vi "close.vi"(0 "reference":refnum<class "OSA.lvclass">, 5 "error in (no error)":errorcluster) -> (19 "error out":errorcluster)   [LabVIEW 2010, in "OSA.lvclass"]
uses:
  OSA.lvclass
  OSA.lvclass/OSA.ctl
  FTSLib.dll
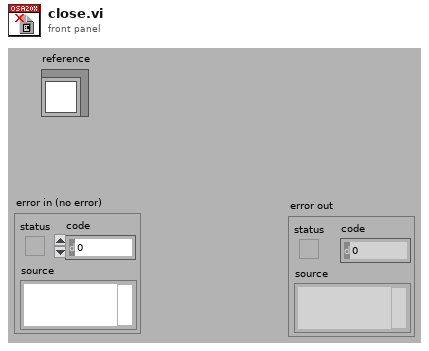
[diagram p1: front panel]
types:
  T1 = typedef "OSA.lvclass/ObjectAttributes.ctl" = cluster{"Stop":bool, "dataType":T2, "spectrometerIdx":u16, "buffer size interferogram":i32, "interferogram":cluster{"new":bool, "plot_x_ min":sgl, "plot_x_max":sgl, "plot_y_min":sgl, "plot_y_max":sgl, "Graph Intrfrgrm":T3, "timeStamp":u32, "signal (%)":dbl, "traces":cluster{"idx":u32, "broadBand":bool, "monoChromatic":bool, "peakToPeakSignal":dbl, "peakToPeakPos":dbl}[], "traces idx last":i32}, "spectrum":cluster{"new":bool, "plot_x_min":sgl, "plot_x_max":sgl, "plot_unit_x":T4, "plot_unit_y":T5, "plot_y_min":sgl, "plot_y_max":sgl, "Graph Spectrum":T3, "timeStamp":u32, "X_VAL_OPTIONS":enum16{"MIN_MAX", "ARRAY"}, "traces":cluster{"idx":u32}[], "traces idx last":i32}, "Thorlabs_OSA_64.lvclass:queue_action.ctlqueue ref":refnum<queue>, "action":T6, "plot zoom step":dbl, "buffer semaphore":T7, "acq stopped":bool, "dataType active":T2, "temperature (degr C)":sgl, "pressure (hPa)":sgl, "rel humidity (%)":sgl, "settings":cluster{"resolution":T8, "sensitivity":T9, "Average":bool, "average nr":u32, "apodisation":T10, "acq delay (ms)":u32, "airMesure":T11, "wmtr on":bool, "intfgrm_smooth_width":u16, "intfgrm_smooth_nrOfPasses":u16, "intfgrm_smooth":T12, "phaseCorrection":T13, "zeroFill":u8, "spectr_smooth":T12, "spectr_smooth_width":u16, "spectr_smooth_nrOfPasses":u16, "resolution (/cm)":sgl, "REF wavelength, (nm)":dbl, "gain_idx":u16, "gainAuto":bool, "gain_relative":dbl, "PD sensitivity mode":T14, "PD senseMode implemented":bool, "SensorTemperature implemented":bool, "SensorPressure implemented":bool, "SensorHumidity implemented":bool}, "peaks position":sgl[], "peaks width":sgl[], "peaks height":sgl[], "peaks max nr":u32, "peaks latest nr":i32, "peaks new":bool, "power":dbl, "power new":bool, "path":string, "wavelength (WNr)":dbl, "wavelength new":bool, "buffer size spectrum":i32, "status":string, "VI reference":refnum<vi>, "funcPointer":u64, "libraryPointer":u64, "singleAcquisition":bool, "coherenceLength (cm)":dbl, "coherenceLength new":bool, "spectrometer model":string, "spectrometer serial nr":string, "peaks thld left":sgl[], "peaks thld right":sgl[], "coherenceLength error (cm)":dbl, "ADC bits":u16, "peaks position centroid":sgl[], "peaks height centroid":sgl[], "OSA series":T15, "channel index (all)":u16}
  T2 = typedef "OSA.lvclass/acq_dataType.ctl" = enum16{"none", "interferogram", "spectrum"}
  T3 = typedef "OSA.lvclass/graph_intensity.ctl" = refnum<vi>
  T4 = typedef "OSA.lvclass/spectrum_x_unit.ctl" = enum16{"wavenr/cm", "THz", "eV", "nm_air", "nm_vac"}
  T5 = typedef "OSA.lvclass/y_unit.ctl" = enum16{"ADC counts", "dBm pwr absolute", "dBm pwr density", "mW pwr absolute", "mW pwr density"}
  T6 = typedef "OSA.lvclass/queue_action.ctl" = enum16{"none", "stop", "GUI_plotInterferogram", "GUI_plotSpectrum", "GUI_plotInterferogramRescale", "GUI_plotSpectrumRescale", "GUI_plotInterferogramReset", "GUI_plotSpectrumReset", "GUI_plotInterferogramAutoScaleY", "GUI_plotSpectrumAutoScaleY", "GUI_plotInterferogramZoomOut", "GUI_plotSpectrumZoomOut", "GUI_plotInterferogramPane", "GUI_plotSpectrumPane", "GUI_plotInterferogramZoomMouse", "GUI_plotSpectrumZoomMouse", "ENVIRONMENT temperature", "ENVIRONMENT pressure", "MODE_resolution set", "MODE_resolution get", "MODE_sensitivity set", "MODE_sensitivity get", "MODE_PDTemperature set", "MODE_PDTemperature get", "REBOOT/RESET firmware", "ACQASYNC_acquireSingleSpectrum", "ACQASYNC_continuous start", "ACQASYNC_continuous stop\n", "ACQASYNC_get last interferogram", "ACQASYNC_get last spectrum", "ACQASYNC_get last waveNr", "ACQOPT_interferogram smoothing set", "ACQOPT_interferogram smoothing get", "ACQOPT_spectrum smoothing set", "ACQOPT_spectrum smoothing get", "ACQOPT_apodisation type set", "ACQOPT_apodisation type get", "ACQOPT_phase correction type set", "ACQOPT_phase correction type get", "ACQOPT_acqIntervall_set", "ACQOPT_acqIntervall_get", "ACQOPT_average spectrum set", "ACQOPT_average spectrum get", "ACQOPT_rolling average set", "ACQOPT_rolling average get", "ACQOPT_zero fill factor set", "ACQOPT_zero fill factor get", "ACQOPT_cycle counting set", "ACQOPT_cycle counting get", "ACQOPT_air measure option set", "ACQOPT_air measure option get", "ACQOPT_gainLevel auto get", "ACQOPT_gainLevel auto set", "ACQOPT_gainLevel get", "ACQOPT_gainLevel set", "ACQOPT_getAll", "INSTRUMENT_PROPERTY_range_WaveNr_min", "INSTRUMENT_PROPERTY_range_WaveNr_max", "INSTRUMENT_PROPERTY_reference_wavelength_cm^-1", "INSTRUMENT_PROPERTY_samplesPerRefPeriod", "INSTRUMENT_PROPERTY_resolution_waveNrPercm", "INSTRUMENT_PROPERTY_availableGainLevels", "INSTRUMENT_PROPERTY_status", "CONVERT", "ANALYSE_POWER", "ANALYSE_PEAKS", "ANALYSE_WAVELENGTH", "ANALYSE_SPECTRUM", "ANALYSE_INTERFEROGRAM", "ANALYSE_COHERENCE_LENGTH", "MATH", "MATH_power", "MATH_peaks", "FILE", "miscellaneous"}
  T7 = typedef "Semaphore RefNum" = refnum<k1>
  T8 = typedef "OSA.lvclass/resolution.ctl" = enum16{"low", "high"}
  T9 = typedef "OSA.lvclass/sensitivityMode.ctl" = enum16{"low", "low medium", "high medium", "high"}
  T10 = typedef "OSA.lvclass/apodisation.ctl" = enum16{"NONE", "NORTON_BEER_WEAK", "NORTON_BEER_MEDIUM", "NORTON_BEER_STRONG", "TRIANGULAR", "COSINE", "HANN", "HAMMING", "BLACKMANHARRIS3", "BLACKMANHARRIS4", "GAUSSIAN"}
  T11 = typedef "OSA.lvclass/airMeasure.ctl" = enum16{"TEMPERATURE", "PRESSURE"}
  T12 = typedef "OSA.lvclass/smoothing.ctl" = enum16{"NONE", "BINOMIAL", "SAVITSKY_GOLAY", "FOURIER", "MOVING_AVERAGE", "GAUSSIAN"}
  T13 = typedef "OSA.lvclass/phaseCorrection.ctl" = enum16{"NONE", "MERTZ", "FORMAN", "MERTZ_FILE", "FORMAN_FILE", "FUTURE COMP."}
  T14 = typedef "OSA.lvclass/PDTemperatureMode.ctl" = enum16{"cool: better sensitivity/noise floor", "warm: extended wl range"}
  T15 = typedef "OSA_series.ctl" = enum16{"OSA200", "OSA300", "UNKNOWN"}
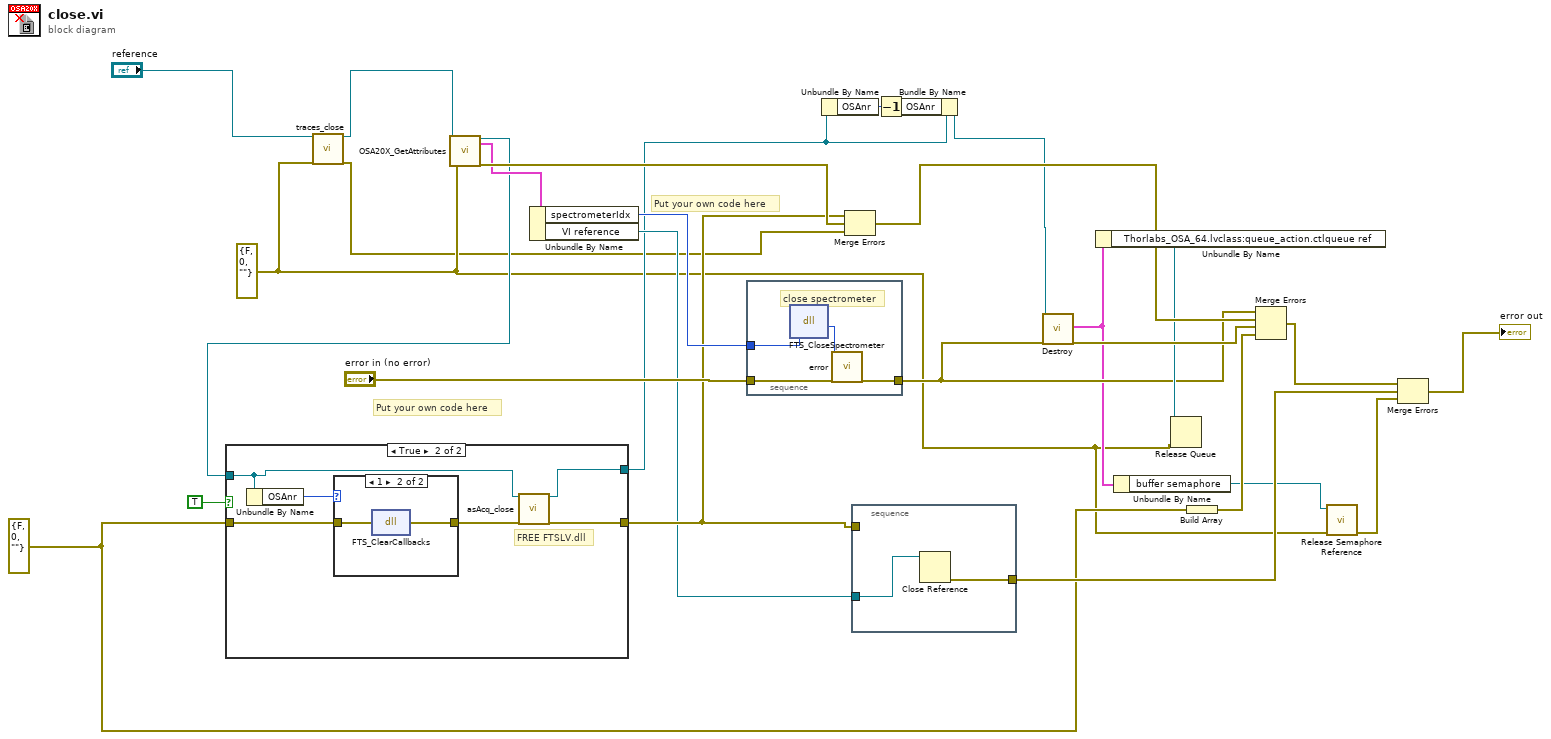
[diagram p0: block diagram]
diagram:
  w15 = errorcluster {"status"=FALSE, "code"=0, "source"=""} ("error in")
  w2 = errorcluster {"status"=FALSE, "code"=0, "source"=""} ("error in (no error)")
  # "Put your own code here"
  # "Put your own code here"
  n1 = call "traces_close.vi"("reference"="reference", "error in (no error)"=w2) -> ("duplicate reference"=w3:refnum<class "OSA.lvclass">, "error out"=w1:errorcluster)  [unwired: 16 in]
  n2 = call "OSA20X_GetAttributes.vi"("reference in"=w3, "error in (no error)"=w2) -> ("reference out"=w12:refnum<class "OSA.lvclass">, "Data"=w14:T1, "error out"=w22:errorcluster)  [unwired: 14 in, 1 out]
  n3 = case shown="True" TRUE {
    tunnel: w12 -> [w30 w31]
    tunnel: [w30 w36] -> w11
    tunnel: [w29 w35] -> w20
    tunnel: w15 -> [w29 w34]
    frame False {
    }
    frame True {
      # "FREE FTSLV.dll"
      n4 = Unbundle By Name(w31) -> ("OSAnr"=w32:i32)
      n5 = case shown="1" w32 {
        tunnel: w34 -> [w37 w39]
        tunnel: [w37 w38] -> w33
        frame 0, Default {
        }
        frame 1 {
          n6 = dll-call lib="FTSLib.dll" fn="FTS_ClearCallbacks"(error in=w39) -> (error out=w38:errorcluster)  [unwired: 3 in, 1 out]
        }
      }
      n7 = call "asAcq_close.vi"("reference"=w31, "error in (no error)"=w33) -> ("duplicate reference"=w36:refnum<class "OSA.lvclass">, "error out"=w35:errorcluster)  [unwired: 16 in]
    }
  }
  n8 = Unbundle By Name(w14) -> ("spectrometerIdx"=w27:u16, "VI reference"=w19:refnum<vi>)
  n9 = stacked-sequence {
    tunnel: "error in (no error)" -> [w42]
    tunnel: w27 -> [w41]
    tunnel: [w40] -> w21
    frame #0 {
      # "close spectrometer"
      n10 = dll-call lib="FTSLib.dll" fn="FTS_CloseSpectrometer"("spectrIdx"=w41) -> ("return type"=w43:i32)  [unwired: 4 in, 2 out]
      n11 = call "error.vi"("result code"=w43, "error in (no error)"=w42) -> ("error out"=w40:errorcluster)  [unwired: 15 in, 2 out]
    }
  }
  n12 = Unbundle By Name(w11) -> ("OSAnr"=w9:i32)
  n13 = Merge Errors(w20, w22, w1) -> (w25:errorcluster)
  n14 = stacked-sequence {
    tunnel: w20 -> [_]
    tunnel: w19 -> [w45]
    tunnel: [w44] -> w18
    frame #0 {
      n15 = Close Reference(reference=w45) -> (error out=w44:errorcluster)  [unwired: 1 in]
    }
  }
  n16 = Decrement(x=w9) -> (x-1=w8:i32)
  n17 = Bundle By Name(cluster=w11, "OSAnr"=w8) -> (w10:refnum<class "OSA.lvclass">)
  n18 = call-dynamic "Destroy.vi"("reference"=w10, "error in (no error)"=w21) -> ("data"=w7:T1, "error out"=w26:errorcluster)  [unwired: 15 in, 1 out]
  n19 = Unbundle By Name(w7) -> ("Thorlabs_OSA_64.lvclass:queue_action.ctlqueue ref"=w24:refnum<queue>)
  n20 = Unbundle By Name(w7) -> ("buffer semaphore"=w6:T7)
  n21 = Release Queue(queue=w24, error in (no error)=w2) -> ()  [unwired: 1 in, 3 out]
  n22 = Build Array(w15) -> (w23:errorcluster[])
  n23 = Merge Errors(w21, w25, w26, w23) -> (w17:errorcluster)
  n24 = call <vilib>:"Release Semaphore Reference.vi"("error in (no error)"=w2, "semaphore"=w6) -> ("error out"=w5:errorcluster)  [unwired: 8 in, 1 out]
  n25 = Merge Errors(w17, w18, w5) -> (→"error out":errorcluster)
